vi "Close_CtlLookup.vi"(8 "error in (no error)":errorcluster, 11 "CtlLookup In":T1) -> (0 "error out":errorcluster)   [LabVIEW 2020, in "CtlReferences.lvlib" / "CtlReferences.lvclass"]
uses:
  CtlReferences.lvclass
  TypeDefs/CtlLookup.ctl
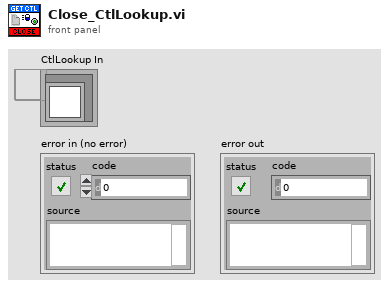
[diagram p1: front panel]
types:
  T1 = typedef "CtlReferences.lvlib/CtlReferences.lvclass/CtlLookup.ctl" = refnum<data-value>
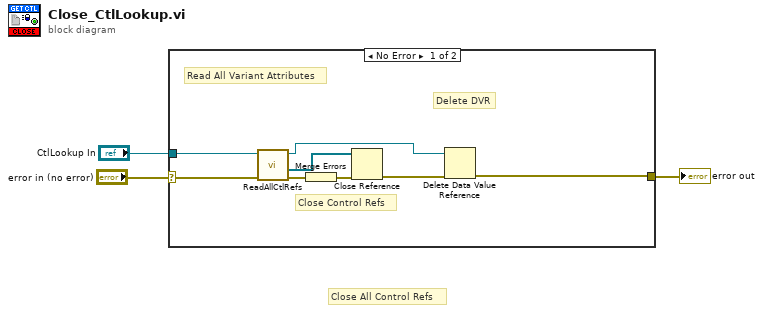
[diagram p0: block diagram]
diagram:
  # "Close All Control Refs"
  n1 = case shown="No Error" "error in (no error)" {
    selector: "error in (no error)" -> [w10 w12]
    tunnel: "CtlLookup In" -> [w9 _]
    tunnel: [w4 w12] -> w2
    frame No Error {
      # "Delete DVR"
      # "Close Control Refs"
      # "Read All Variant Attributes"
      n2 = call "ReadAllCtlRefs.vi"("error in (no error)"=w10, "CtlLookup In"=w9) -> ("error out"=w8:errorcluster, "CtlRef Array"=w7:refnum<vi>[], "CtlLookup Out"=w5:T1)  [unwired: 6 in, 1 out]
      n3 = Merge Errors(w8) -> (w11:errorcluster)
      n4 = Close Reference(reference=w7, error in (no error)=w11) -> (error out=w6:errorcluster)
      n5 = Delete Data Value Reference(data value reference=w5, error in=w6) -> (error out=w4:errorcluster)  [unwired: 1 out]
    }
    frame Error {
    }
  }
  "error out" <- w2
